vi "update system version in config.vi"(8 "error in":errorcluster, 10 "version":T1, 11 "shared memory editor node":refnum<class "module editor node.lvclass">) -> (0 "error out":errorcluster, 3 "shared memory editor node out":refnum<class "module editor node.lvclass">)   [LabVIEW 2014, in "Shared Memory editor node.lvclass"]
uses:
  Shared Memory editor node.lvclass
  <vilib>/NI/DCAF/Tag Editor Core/Configuration Editor/Classes/Module editor node/module editor node.lvclass
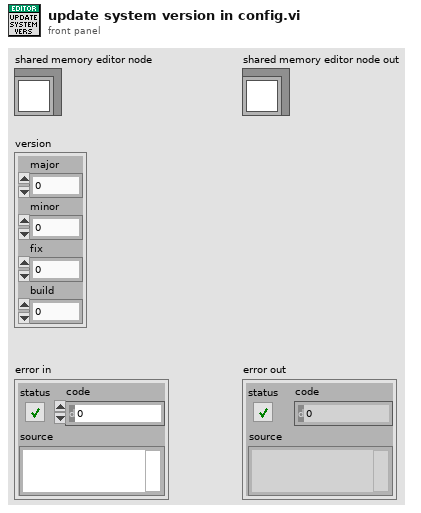
[diagram p1: front panel]
types:
  T1 = cluster{"major":u16, "minor":u16, "fix":u16, "build":u16}
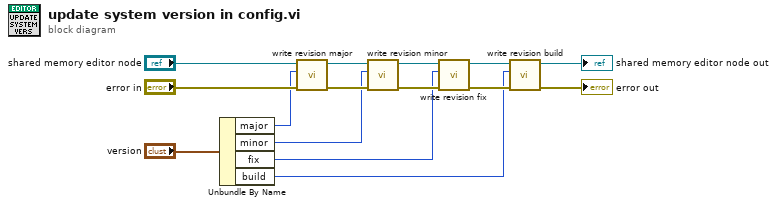
[diagram p0: block diagram]
diagram:
  n1 = Unbundle By Name("version") -> ("major"=w4:u16, "minor"=w3:u16, "fix"=w2:u16, "build"=w1:u16)
  n2 = call "write revision major.vi"("error in"="error in", "revision major"=w4, "shared memory editor node"="shared memory editor node") -> ("error out"=w8:errorcluster, "shared memory editor node out"=w12:refnum<class "module editor node.lvclass">)  [unwired: 7 in]
  n3 = call "write revision minor.vi"("error in"=w8, "revision minor"=w3, "shared memory editor node"=w12) -> ("error out"=w7:errorcluster, "shared memory editor node out"=w11:refnum<class "module editor node.lvclass">)  [unwired: 7 in]
  n4 = call "write revision fix.vi"("error in"=w7, "revision fix"=w2, "shared memory editor node"=w11) -> ("error out"=w6:errorcluster, "shared memory editor node out"=w10:refnum<class "module editor node.lvclass">)  [unwired: 7 in]
  n5 = call "write revision build.vi"("error in"=w6, "revision build"=w1, "shared memory editor node"=w10) -> ("error out"=→"error out":errorcluster, "shared memory editor node out"=→"shared memory editor node out":refnum<class "module editor node.lvclass">)  [unwired: 7 in]
